vi "ClientSrv Digest Password.vi"(0 "server name (none)":string, 7 "password":string, 11 "static salt (default)":string="¼lPJõ_|\u0003š–!ä") -> (8 "SHA-1 digest":string)   [LabVIEW 2012]
doc: "Combines the server name, a password, and some static salt and calculates a SHA-1 digest. By transferring the digest instead of the plain-text password for verification over the network, security is improved.\n\nThe remainder of the diagram implements the Secure Hash Algorithm (SHA-1) for computing a condensed representation of a message or a data file, as specified in FIPS PUB 180-1, Secure Hash Standard (see note below).\n\nWhen a message of any length < 2^64 (see note below) is input, the SHA-1 produces a 160-bit output called a message digest. The SHA-1 is called secure because it is computationally infeasible to find a message which correspond to a given message digest, or to find two different messages which produce the same digest.\n\n<B>Note:</B> No independent assertion of the security of this hash function by the authors for any particular use is intended.\n\nAlthough the SHA-1 is valid for messages with length < 2^64, this implementation is limited to messages < 2^32."
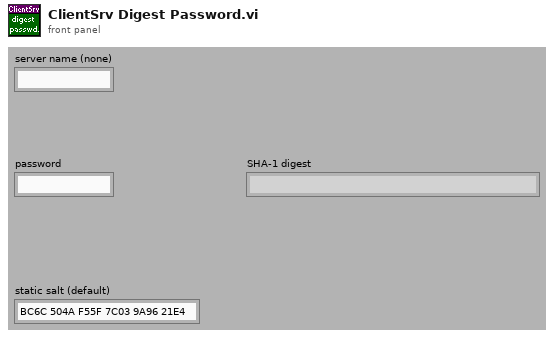
[diagram p1: front panel]
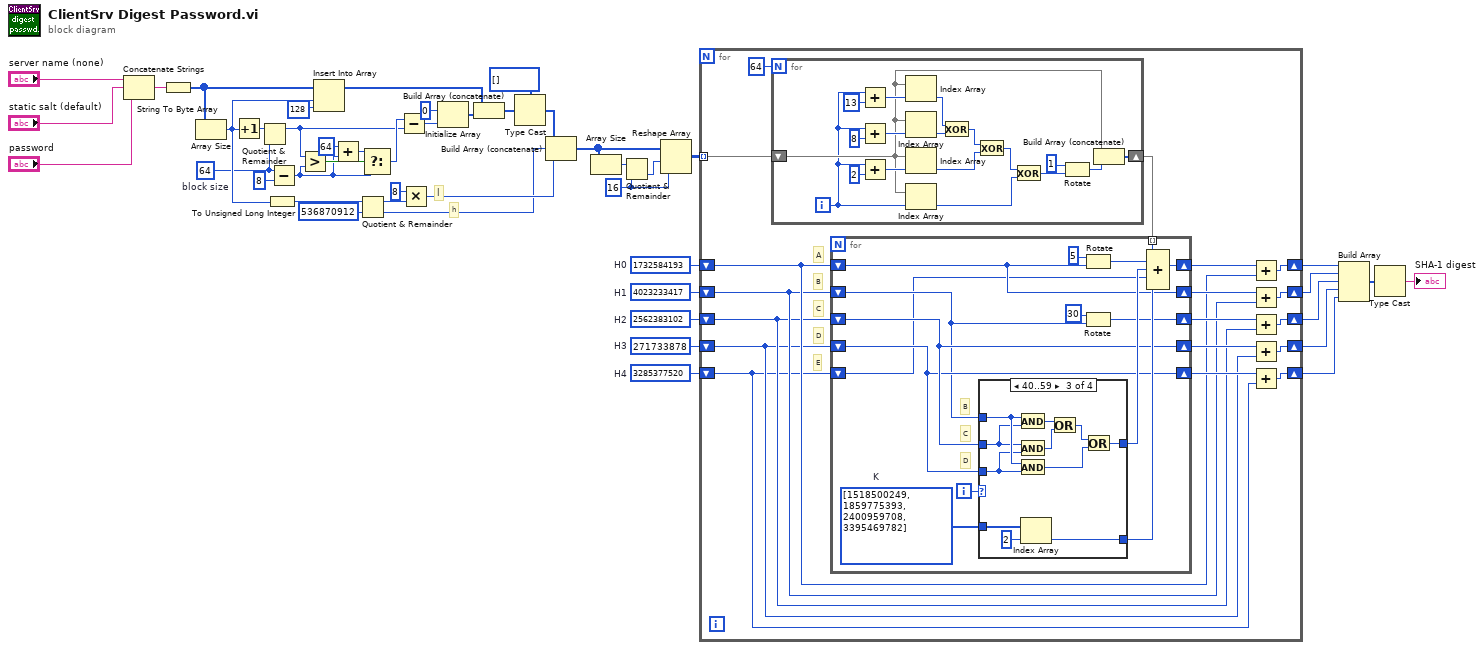
[diagram p0: block diagram]
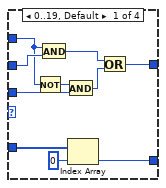
[diagram p2: hidden frame]
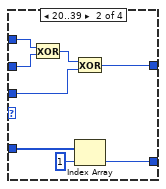
[diagram p3: hidden frame]
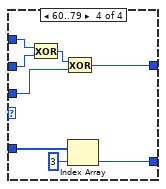
[diagram p4: hidden frame]
diagram:
  w7 = 64  # block size
  w32 = 16 ("y")
  w42 = u32 3285377520  # H4
  w43 = u32 271733878  # H3
  w44 = u32 2562383102  # H2
  w45 = u32 4023233417  # H1
  w46 = u32 1732584193  # H0
  # "h"
  # "l"
  n1 = Concatenate Strings("server name (none)", "static salt (default)", "password") -> (w4:string)
  n2 = String To Byte Array(string=w4) -> (unsigned byte array=w6:u8[])
  n3 = Array Size(array=w6) -> (size(s)=w11:i32)
  n4 = Increment(x=w11) -> (x+1=w28:i32)
  n5 = Quotient & Remainder(x=w28, y=w7) -> (x-y*floor(x/y)=w21:i32)  [unwired: 1 out]
  n6 = To Unsigned Long Integer(number=w11) -> (unsigned 32bit integer=w12:u32)
  n7 = Subtract(x=w7, y=8) -> (x-y=w17:i32)
  n8 = Greater?(x=w21, y=w17) -> (0:w23:bool)
  n9 = Insert Into Array(array=w6, index=w11, new element=u8 128 ("Element Data")) -> (w27:u8[])
  n10 = Add(x=64 ("y"), y=w17) -> (x+y=w19:i32)
  n11 = Quotient & Remainder(x=w12, y=u32 536870912) -> (x-y*floor(x/y)=w10:u32, floor(x/y)=w8:u32)
  n12 = Select(t=w19, s=w23, f=w17) -> (s? t:f=w22:i32)
  n13 = Subtract(x=w22, y=w21) -> (x-y=w25:i32)
  n14 = Multiply(x=u32 8, y=w10) -> (x*y=w9:u32)
  n15 = Initialize Array(u8 0 ("Element Data"), w25) -> (w24:u8[])
  n16 = Build Array (concatenate)(w27, w24) -> (w15:u8[])
  n17 = Type Cast(type=u32[] [], x=w15) -> (*(type *) &x=w14:u32[])
  n18 = Build Array (concatenate)(w14, w8, w9) -> (w5:u32[])
  n19 = Array Size(array=w5) -> (size(s)=w33:i32)
  n20 = Quotient & Remainder(x=w33, y=w32) -> (floor(x/y)=w31:i32)  [unwired: 1 out]
  n21 = Reshape Array(w5, w31, w32) -> (w34:u32[][])
  n22 = for {
    tunnel: w34 -> [w64] mode=indexing
    shift-right: [w63] -> w41
    shift-left: w46 -> [w53]
    shift-right: [w62] -> w40
    shift-left: w45 -> [w52]
    shift-right: [w61] -> w39
    shift-left: w44 -> [w51]
    shift-right: [w60] -> w38
    shift-left: w43 -> [w50]
    shift-right: [w59] -> w37
    shift-left: w42 -> [w49]
    # "A"
    # "B"
    # "C"
    # "D"
    # "E"
    n23 = for {
      N: 64 -> [_]
      shift-right: [w120] -> w48
      shift-left: w64 -> [w121]
      i -> [w117]
      n24 = Add(x=w117, y=13) -> (x+y=w134:i32)
      n25 = Add(x=w117, y=8) -> (x+y=w132:i32)
      n26 = Add(x=w117, y=2) -> (x+y=w133:i32)
      n27 = Index Array(array=w121, index=w134) -> (element=w128:u32)
      n28 = Index Array(array=w121, index=w132) -> (element=w127:u32)
      n29 = Index Array(array=w121, index=w133) -> (element=w125:u32)
      n30 = Index Array(array=w121, index=w117) -> (element=w123:u32)
      n31 = Exclusive Or(1:w127, 2:w128) -> (0:w126:u32)
      n32 = Exclusive Or(1:w125, 2:w126) -> (0:w124:u32)
      n33 = Exclusive Or(1:w123, 2:w124) -> (0:w122:u32)
      n34 = Rotate(1:w122, 2:i8 1 ("n")) -> (0:w119:u32)
      n35 = Build Array (concatenate)(w121, w119) -> (w120:u32[])
    }
    n36 = for {
      tunnel: w48 -> [w77] mode=indexing
      shift-right: [w72] -> w58
      shift-left: w53 -> [w70]
      shift-right: [w70] -> w57
      shift-left: w52 -> [w68]
      shift-right: [w66] -> w56
      shift-left: w51 -> [w74]
      shift-right: [w74] -> w55
      shift-left: w50 -> [w73]
      shift-right: [w73] -> w54
      shift-left: w49 -> [w65]
      i -> [w78]
      w79 = u32[] [1518500249, 1859775393, 2400959708, 3395469782]  # K
      # "D"
      # "C"
      # "B"
      n37 = case shown="40..59" w78 {
        tunnel: w68 -> [w85 w95 w106 w112]
        tunnel: w74 -> [w87 w94 w105 w111]
        tunnel: w73 -> [w84 w92 w104 w110]
        tunnel: w79 -> [w89 w97 w108 w116]
        tunnel: [w81 w91 w99 w113] -> w76
        tunnel: [w80 w90 w98 w109] -> w75
        frame 0..19, Default {
          n38 = Not(x=w85) -> (.not. x?=w86:u32)
          n39 = And(x=w85, y=w87) -> (x .and. y?=w83:u32)
          n40 = And(x=w86, y=w84) -> (x .and. y?=w82:u32)
          n41 = Index Array(array=w89, index=0 ("Index")) -> (element=w80:u32)
          n42 = Or(x=w83, y=w82) -> (x .or. y?=w81:u32)
        }
        frame 20..39 {
          n43 = Exclusive Or(1:w94, 2:w95) -> (0:w93:u32)
          n44 = Exclusive Or(1:w92, 2:w93) -> (0:w91:u32)
          n45 = Index Array(array=w97, index=1 ("Index")) -> (element=w90:u32)
        }
        frame 40..59 {
          n46 = And(x=w106, y=w105) -> (x .and. y?=w103:u32)
          n47 = And(x=w105, y=w104) -> (x .and. y?=w102:u32)
          n48 = And(x=w106, y=w104) -> (x .and. y?=w100:u32)
          n49 = Index Array(array=w108, index=2 ("Index")) -> (element=w98:u32)
          n50 = Or(x=w103, y=w102) -> (x .or. y?=w101:u32)
          n51 = Or(x=w101, y=w100) -> (x .or. y?=w99:u32)
        }
        frame 60..79 {
          n52 = Exclusive Or(1:w111, 2:w112) -> (0:w114:u32)
          n53 = Exclusive Or(1:w110, 2:w114) -> (0:w113:u32)
          n54 = Index Array(array=w116, index=3 ("Index")) -> (element=w109:u32)
        }
      }
      n55 = Rotate(1:w70, 2:i8 5 ("n")) -> (0:w69:u32)
      n56 = Rotate(1:w68, 2:i8 30 ("n")) -> (0:w66:u32)
      n57 = Compound Arithmetic op=ADD(w77, w69, w76, w65, w75) -> (w72:u32)
    }
    n58 = Add(x=w58, y=w53) -> (x+y=w63:u32)
    n59 = Add(x=w57, y=w52) -> (x+y=w62:u32)
    n60 = Add(x=w56, y=w51) -> (x+y=w61:u32)
    n61 = Add(x=w55, y=w50) -> (x+y=w60:u32)
    n62 = Add(x=w54, y=w49) -> (x+y=w59:u32)
  }
  n63 = Build Array(w41, w40, w39, w38, w37) -> (w36:u32[])
  n64 = Type Cast(x=w36) -> (*(type *) &x=→"SHA-1 digest":string)  [unwired: 1 in]
